vi "moveLogic.vi"(2 "distanceThreshold":dbl=0.1, 3 "nextPos":cluster{"x":dbl, "y":dbl}, 4 "robotPos":cluster{"x":dbl, "y":dbl, "theta":dbl}) -> (0 "arrived?":bool=TRUE, 1 "outputSpeed":cluster{"left":dbl, "right":dbl}={"left"=1.0, "right"=-1.0})   [LabVIEW 2016]
panel:
  in  "speedTemplate":cluster{"left":dbl, "right":dbl}={"left"=1.0, "right"=-1.0}
  out "String":string
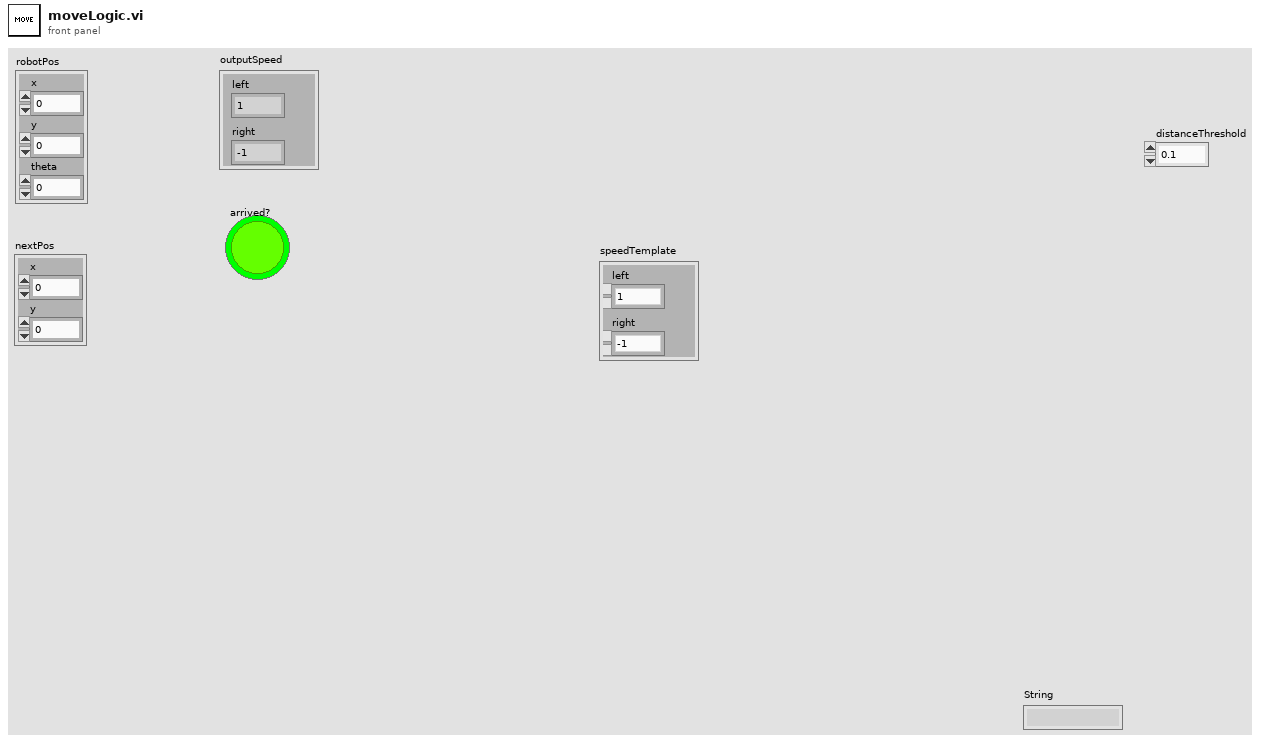
[diagram p1: front panel]
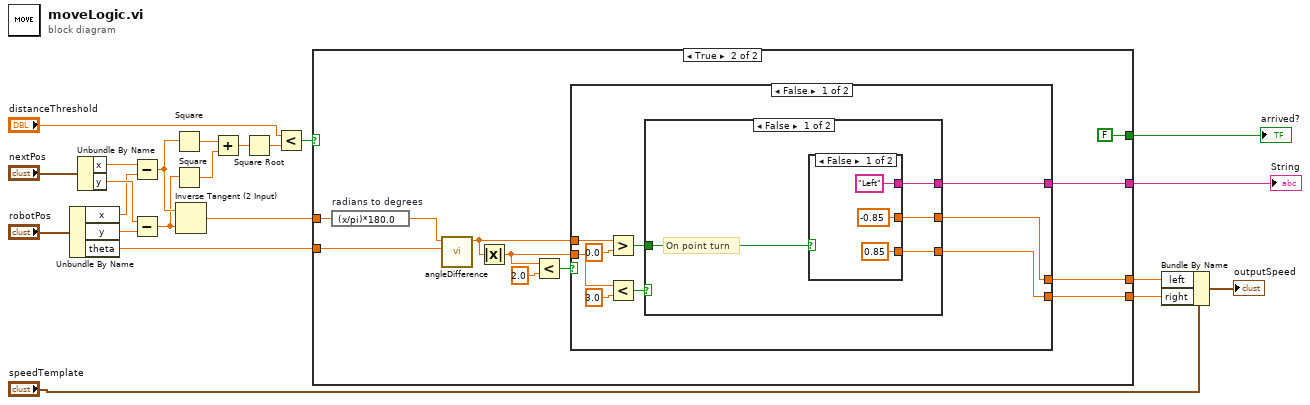
[diagram p0: block diagram]
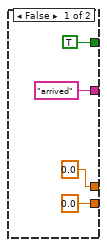
[diagram p2: hidden frame]
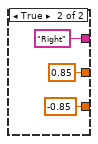
[diagram p3: hidden frame]
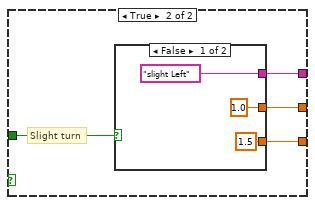
[diagram p4: hidden frame]
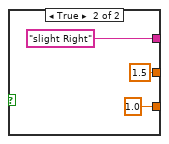
[diagram p5: hidden frame]
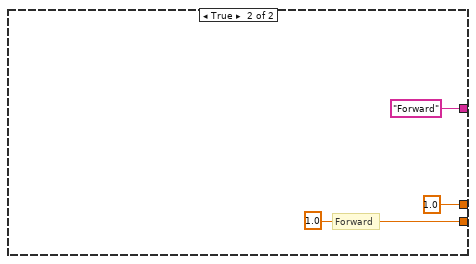
[diagram p6: hidden frame]
diagram:
  n1 = Unbundle By Name("robotPos") -> ("x"=w6:dbl, "y"=w5:dbl, "theta"=w4:dbl)
  n2 = Unbundle By Name("nextPos") -> ("x"=w9:dbl, "y"=w8:dbl)
  n3 = Subtract(x=w9, y=w6) -> (x-y=w2:dbl)
  n4 = Subtract(x=w8, y=w5) -> (x-y=w1:dbl)
  n5 = Square(x=w2) -> (x^2=w17:dbl)
  n6 = Square(x=w1) -> (x^2=w18:dbl)
  n7 = Inverse Tangent (2 Input)(1:w1, 2:w2) -> (0:w19:dbl)
  n8 = Add(x=w17, y=w18) -> (x+y=w16:dbl)
  n9 = Square Root(x=w16) -> (sqrt(x)=w15:dbl)
  n10 = Less?(x="distanceThreshold", y=w15) -> (x < y?=w20:bool)
  n11 = case shown="True" w20 {
    tunnel: [0.0 w32] -> w11
    tunnel: [0.0 w31] -> w13
    tunnel: [TRUE FALSE] -> w22
    tunnel: w19 -> [_ w36]
    tunnel: w4 -> [_ w28]
    tunnel: ["arrived" ("String") w27] -> w3
    frame False {
    }
    frame True {
      n12 = expression code="(x/pi)*180.0" "radians to degrees"(w36) -> (w30:dbl)
      n13 = call "angleDifference.vi"("theta B"=w28, "theta A"=w30) -> ("delta theta"=w29:dbl)  [unwired: 9 in]
      n14 = Absolute Value(x=w29) -> (abs(x)=w33:dbl)
      n15 = Less?(x=w33, y=2.0) -> (x < y?=w35:bool)
      n16 = case shown="False" w35 {
        tunnel: w33 -> [w46 _]
        tunnel: [w42 1.0] -> w32
        tunnel: [w43 1.0] -> w31
        tunnel: w29 -> [w39 _]
        tunnel: [w38 "Forward" ("String")] -> w27
        frame False {
          n17 = Greater?(x=w39, y=0.0) -> (0:w40:bool)
          n18 = Less?(x=w46, y=3.0) -> (x < y?=w44:bool)
          n19 = case shown="False" w44 {
            tunnel: [w50 w60] -> w43
            tunnel: [w49 w59] -> w42
            tunnel: w40 -> [w48 w58]
            tunnel: [w47 w57] -> w38
            frame False {
              # "On point turn"
              n20 = case shown="False" w48 {
                tunnel: [-0.85 0.85] -> w50
                tunnel: [0.85 -0.85] -> w49
                tunnel: ["Left" ("String") "Right" ("String")] -> w47
                frame False {
                }
                frame True {
                }
              }
            }
            frame True {
              # "Slight turn"
              n21 = case shown="False" w58 {
                tunnel: [1.0 1.5] -> w60
                tunnel: [1.5 1.0] -> w59
                tunnel: ["slight Left" ("String") "slight Right" ("String")] -> w57
                frame False {
                }
                frame True {
                }
              }
            }
          }
        }
        frame True {
          # "Forward"
        }
      }
    }
  }
  "arrived?" <- w22
  "String" <- w3
  n22 = Bundle By Name(cluster="speedTemplate", "left"=w13, "right"=w11) -> (→"outputSpeed":cluster{"left":dbl, "right":dbl})
